vi "BuildTestFromProjectItem_LibraryWithPrivateMember_BuildsEmptyTestSuite.vi"() -> ()   [LabVIEW 2017, in "LVUnitTestBuilder.Tests.lvlib"]
uses:
  LVUnitTestBuilder.Tests.lvlib
  LVUnitTestBuilder/LVUnitTestBuilder.lvclass
  TestSuite/TestSuite.lvclass
  a12a2084-e44a-4edc-a973-f21fdd0e5ac6.vi
  Constraint/IsEqual/Create.vi
  Constraint/IsEqual/IsEqual.lvclass
panel:
  out "error out":errorcluster
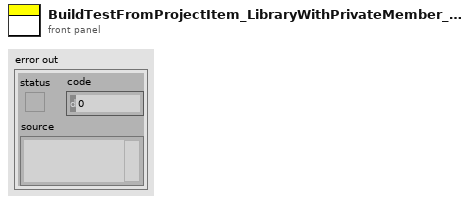
[diagram p1: front panel]
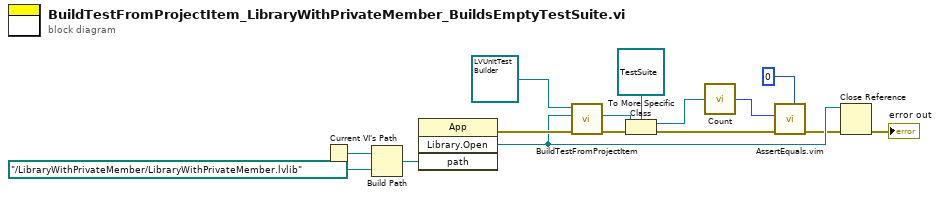
[diagram p0: block diagram]
diagram:
  n1 = Current VI's Path() -> (path=w2:path)
  n2 = Build Path(base path=w2, name or relative path=path "../LibraryWithPrivateMember/LibraryWithPrivateMember.lvlib") -> (appended path=w1:path)
  n3 = invoke class="App" method="Library.Open"("path"=w1) -> (error out=w14:errorcluster, "Open Library"=w9:refnum<vi>)  [unwired: 3 in, 2 out]
  n4 = call-dynamic "BuildTestFromProjectItem.vi"("error in (no error)"=w14, "ProjectItem Refnum"=w9, "LVUnitTestBuilder in"=refnum<class "LVUnitTestBuilder.lvclass"> refnum ("LVUnitTestBuilder")) -> ("error out"=w8:errorcluster, "Test"=w13:refnum<class "Test.lvclass">)  [unwired: 6 in, 1 out]
  n5 = To More Specific Class(target class=refnum<class "TestSuite.lvclass"> refnum ("TestSuite.lvclass"), reference=w13, error in=w8) -> (specific class reference=w11:refnum<class "TestSuite.lvclass">, error out=w7:errorcluster)
  n6 = call "Count.vi"("TestSuite In"=w11) -> ("Count"=w5:i32)
  n7 = call "AssertEquals.vim"("Expected"=0 ("Count"), "error in (no error)"=w7, "Actual"=w5) -> ("error out"=w6:errorcluster)  [unwired: 8 in]
  n8 = Close Reference(reference=w9, error in (no error)=w6) -> (error out=→"error out":errorcluster)
